vi "Contains.vi"(5 "Invert?":bool, 10 "y":string, 11 "x":string) -> (2 "Equal?":bool)   [LabVIEW 2018]
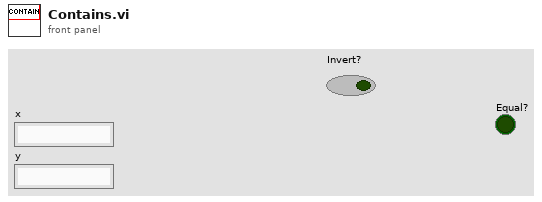
[diagram p1: front panel]
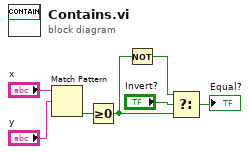
[diagram p0: block diagram]
diagram:
  n1 = Match Pattern(string="x", regular expression="y") -> (offset past match=w2:i32)  [unwired: 1 in, 3 out]
  n2 = Greater Or Equal To 0?(x=w2) -> (x >= 0?=w1:bool)
  n3 = Not(x=w1) -> (.not. x?=w6:bool)
  n4 = Select(t=w6, s="Invert?", f=w1) -> (s? t:f=→"Equal?":bool)
